vi "MQTT HASS Publisher.vi"() -> ()   [LabVIEW 2021]
uses:
  <vilib>/LabVIEW Open Source Project/MQTT Control Packets/Control Packets/CONNECT/ConnectFlags -- cluster.ctl
  <vilib>/LabVIEW Open Source Project/MQTT Connection/MQTT_Base/Base Class/MQTT_Base.lvclass/MQTT_Base.ctl
  <vilib>/LabVIEW Open Source Project/Connection/Connection.TCP/Connection.TCP.lvclass
  C:/Program Files (x86)/National Instruments/LabVIEW 2021/vi.lib/LabVIEW Open Source Project/Connection/Connection/Connection.lvclass
  <vilib>/LabVIEW Open Source Project/MQTT Client/Client class/Client.lvclass
  C:/Program Files (x86)/National Instruments/LabVIEW 2021/vi.lib/LabVIEW Open Source Project/MQTT Connection/MQTT_Base/Base Class/MQTT_Base.lvclass
  <vilib>/LabVIEW Open Source Project/MQTT Control Packets/Control Packets/PUBLISH/PUBLISH.lvclass
  <vilib>/LabVIEW Open Source Project/MQTT Connection/MQTT_Base/Base Class/MQTT_Base.lvclass
  <vilib>/LabVIEW Open Source Project/MQTT Control Packets/Control Packets/CONNECT/CONNECT.lvclass
  <vilib>/LabVIEW Open Source Project/MQTT Control Packets/Control Packets/ControlPacket/ControlPacket.lvclass
panel:
  out "Config Topic":string
  out "Voltage chart":dbl(graph)
  in  "Time Target (s)":dbl=0.5 format="%#_6ps"
  out "Current Chart":dbl(graph)
  out "State String":string
  out "Published State":bool
  in  "State topic":string="lab/psu/state"
  in  "Send Config Btn":bool
  out "Config String":string
  out "Connected?":bool
  out "Published Config":bool
  in  "remote port (1883)":u16=1883
  in  "address (localhost)":string="localhost"
  in  "STOP":bool
  # "HASS Publisher"
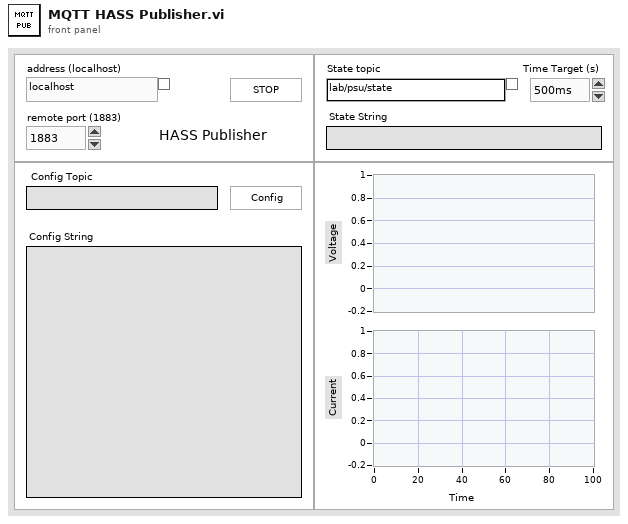
[diagram p1: front panel]
types:
  T1 = cluster{"Topic Name":string, "Config Message":string}[]
  T2 = enum32{"Invalid", "Standard", "Closed", "Hidden", "Minimized", "Maximized"}
  T3 = enum32{"invalid app kind", "Development System", "Run Time System", "Student Edition", "Embedded LabVIEW", "Evaluation", "Custom"}
  T4 = typedef "MQTT_Control_Packets.lvlib/CONNECT.lvclass/ConnectFlags -- cluster.ctl" = cluster{"Reserved":bool, "Clean Session":bool, "Will Flag":bool, "Will QoS 1":bool, "Will QoS 2":bool, "Will Retain":bool, "Password Flag":bool, "User Name Flag":bool}
  T5 = cluster{"Will Topic":string, "Will Message":string, "Username":string, "Password":string}
  T6 = cluster{"Core":cluster{"Current VI Reference":refnum<vi>, "Close Panel on Exit?":bool}, "Connected?":bool, "Published Config?":bool, "Published State?":bool, "Voltage":dbl, "Current":dbl}
  T7 = cluster{"Current VI Reference":refnum<vi>, "Close Panel on Exit?":bool}
  T8 = typedef "MQTT Base.lvlib/MQTT_Base.lvclass/Public Events -- cluster.ctl" = cluster{"Stop Event":refnum<user-event>, "Error Event":refnum<user-event>, "Inbound Message":refnum<user-event>}
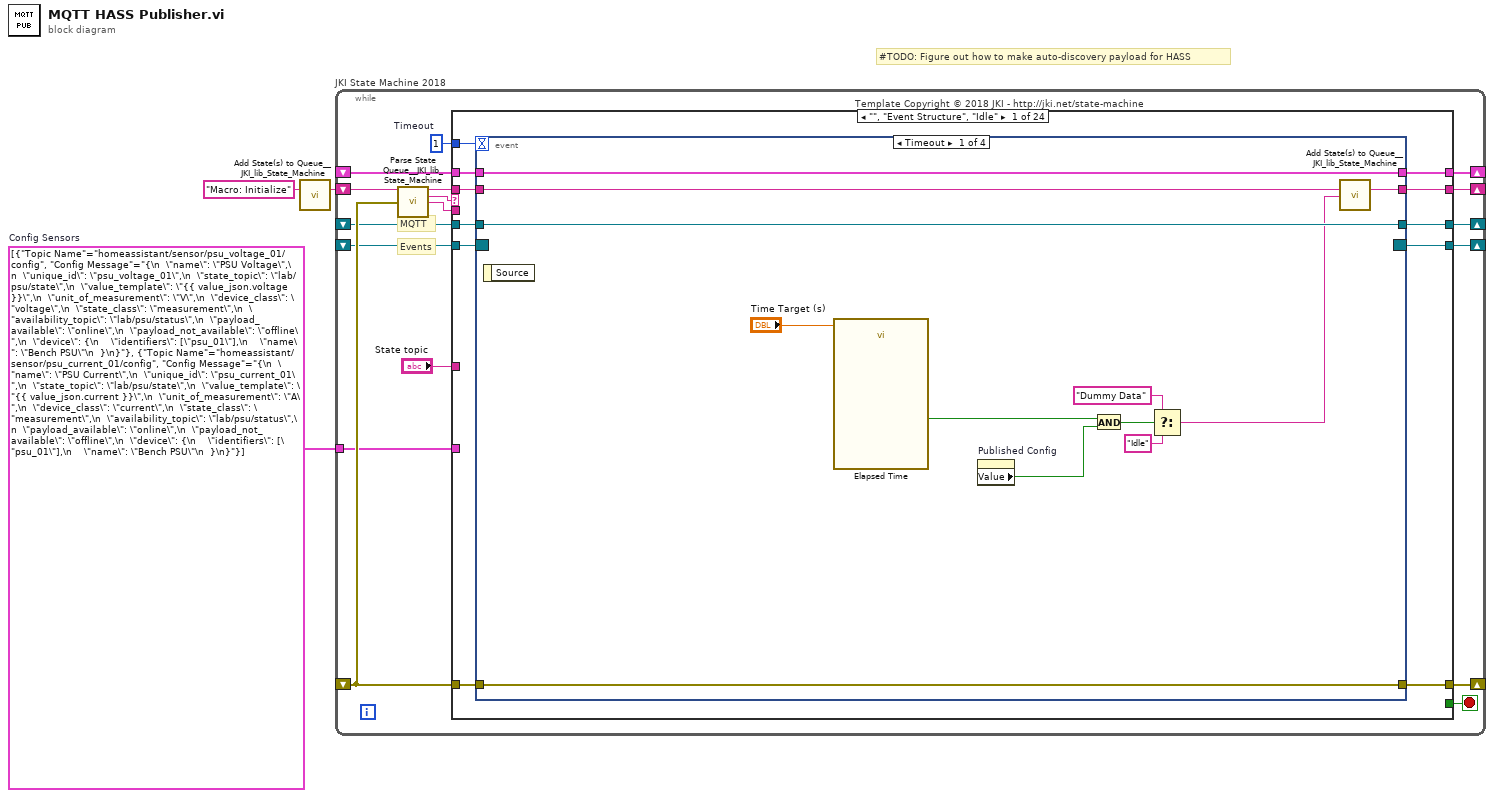
[diagram p0: block diagram]
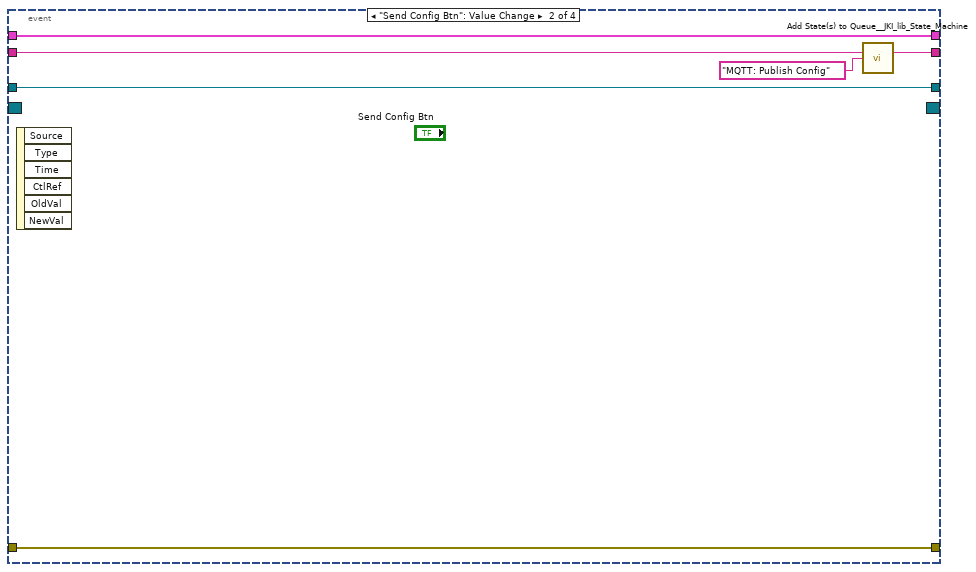
[diagram p2: hidden frame]
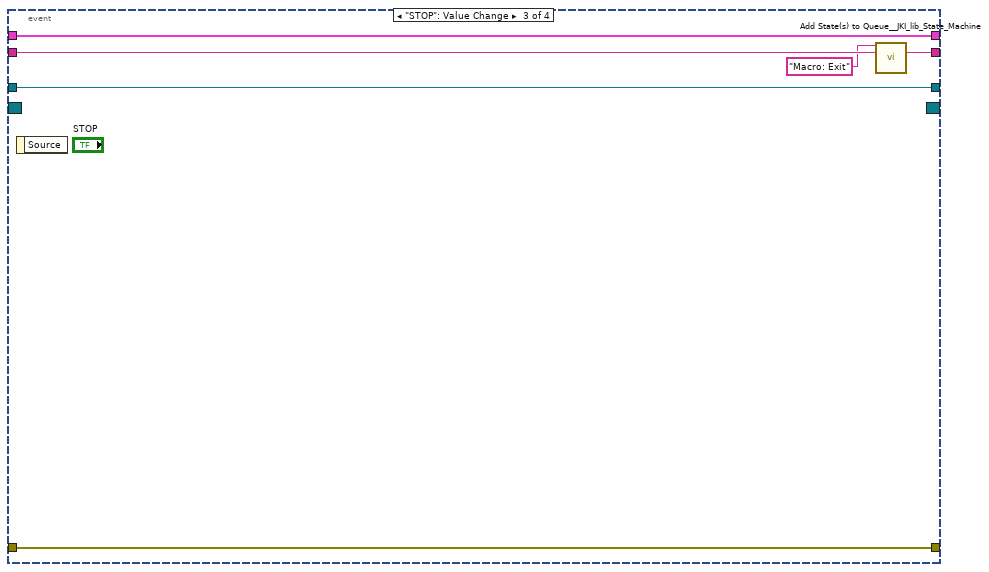
[diagram p3: hidden frame]
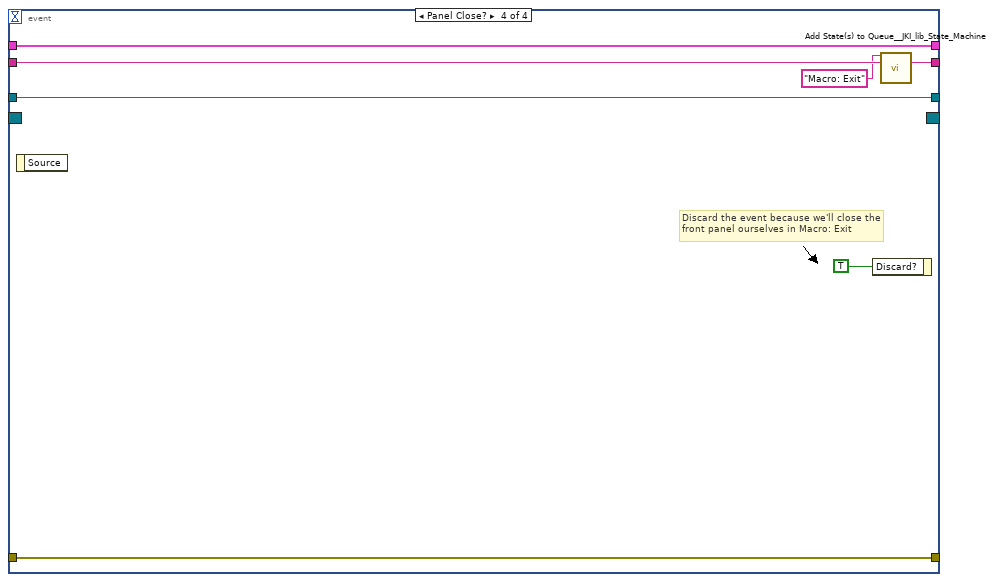
[diagram p4: hidden frame]
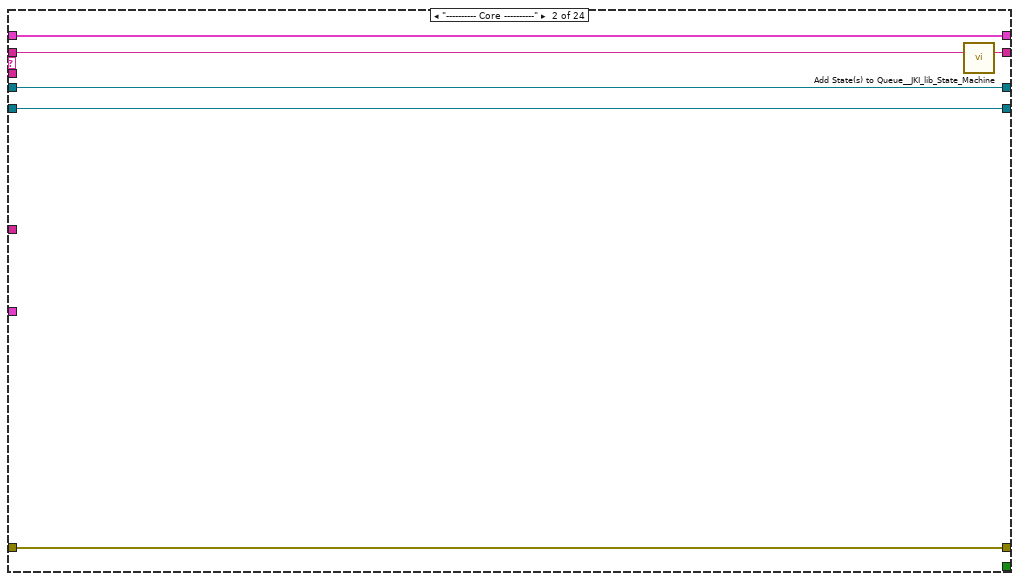
[diagram p5: hidden frame]
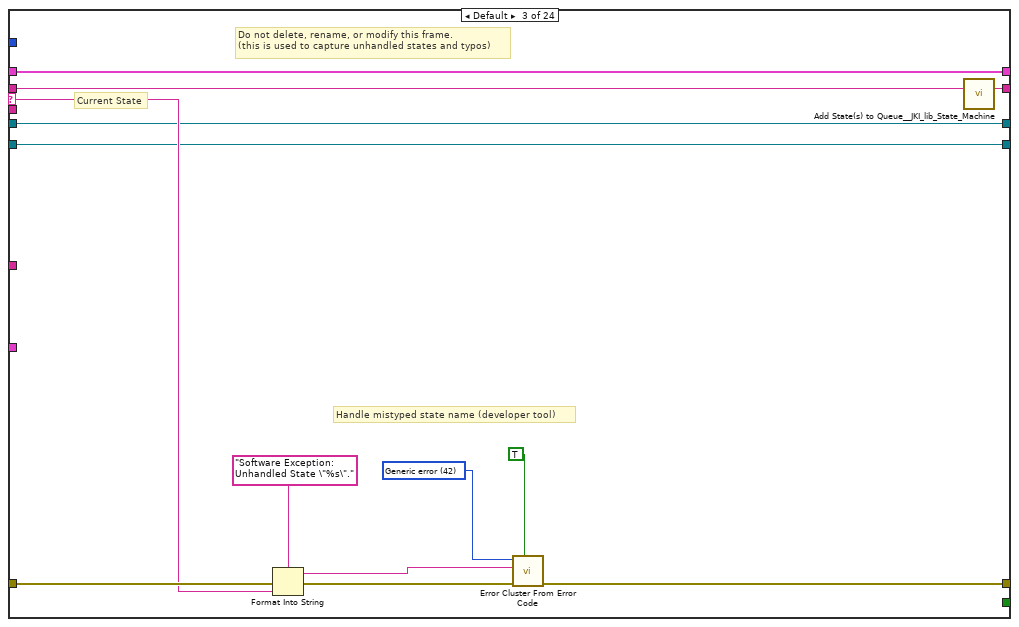
[diagram p6: hidden frame]
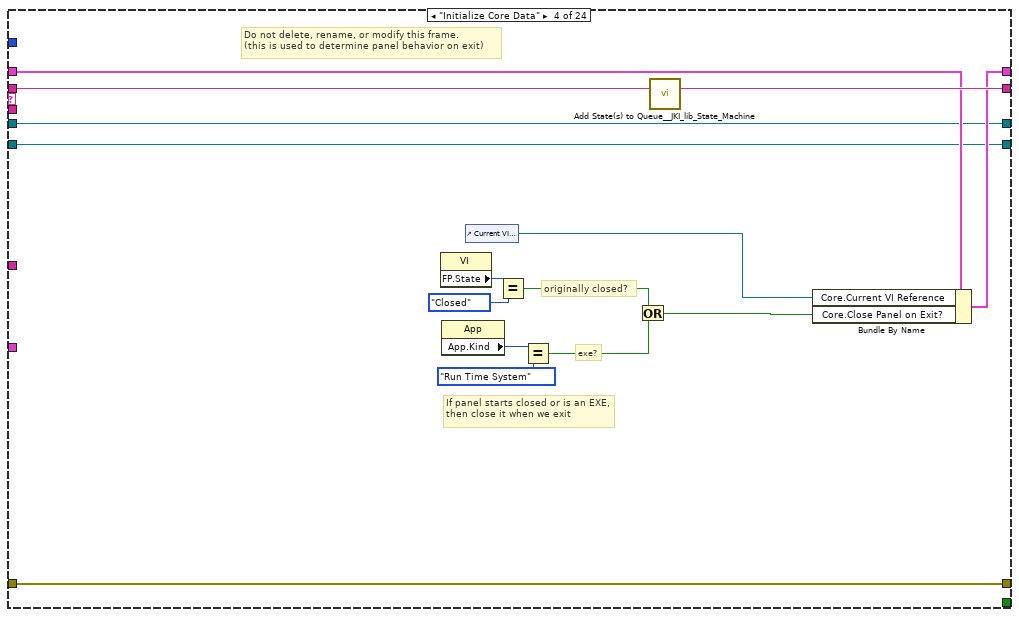
[diagram p7: hidden frame]
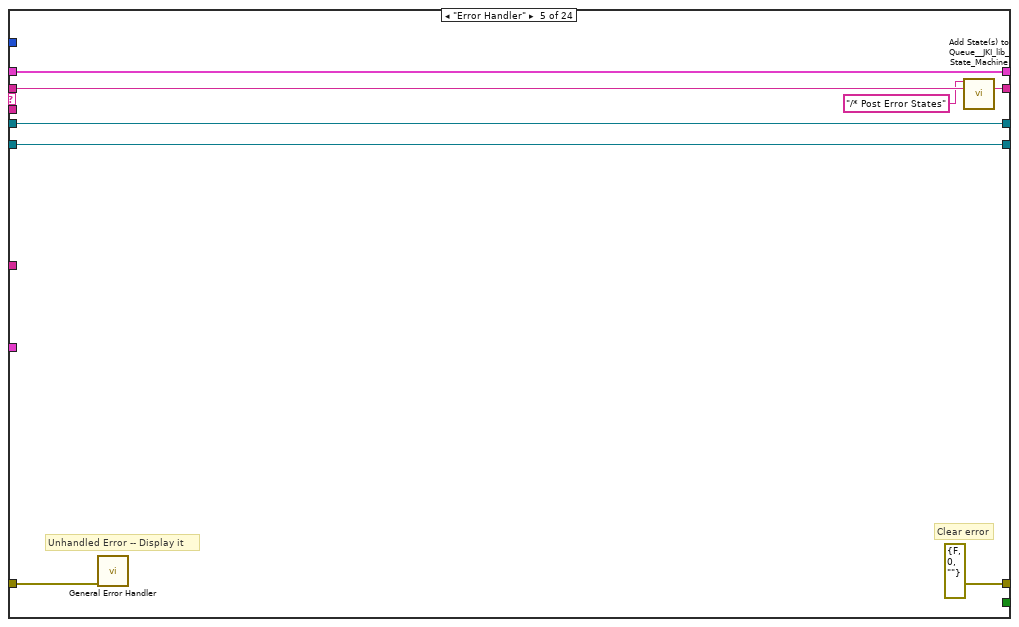
[diagram p8: hidden frame]
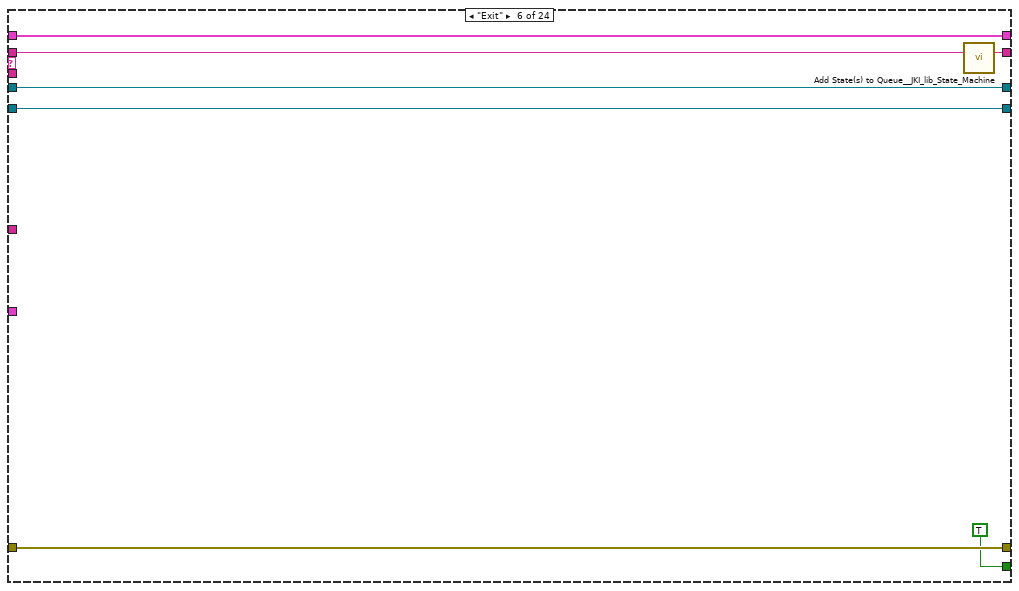
[diagram p9: hidden frame]
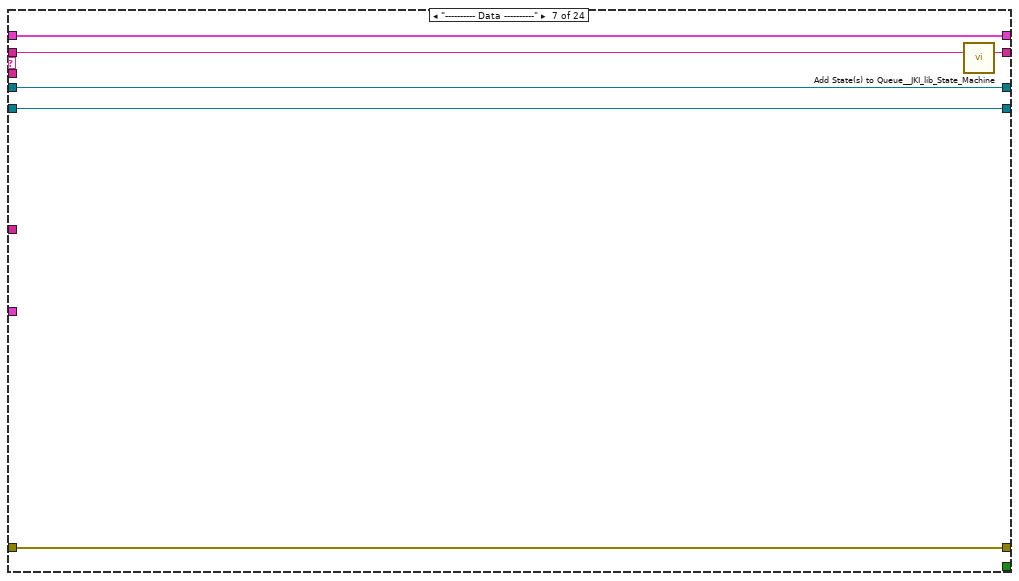
[diagram p10: hidden frame]
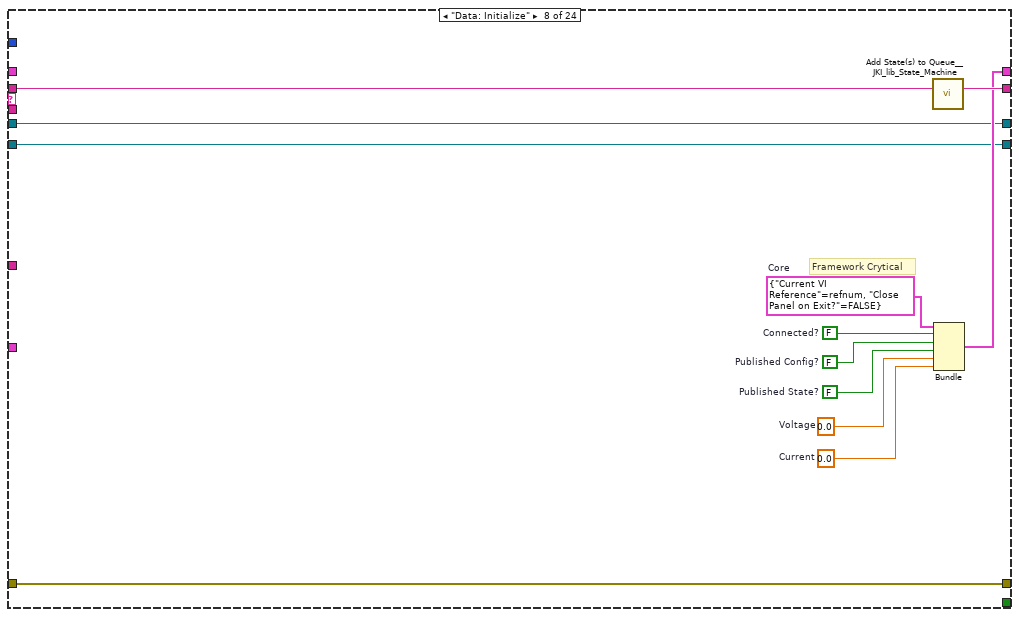
[diagram p11: hidden frame]
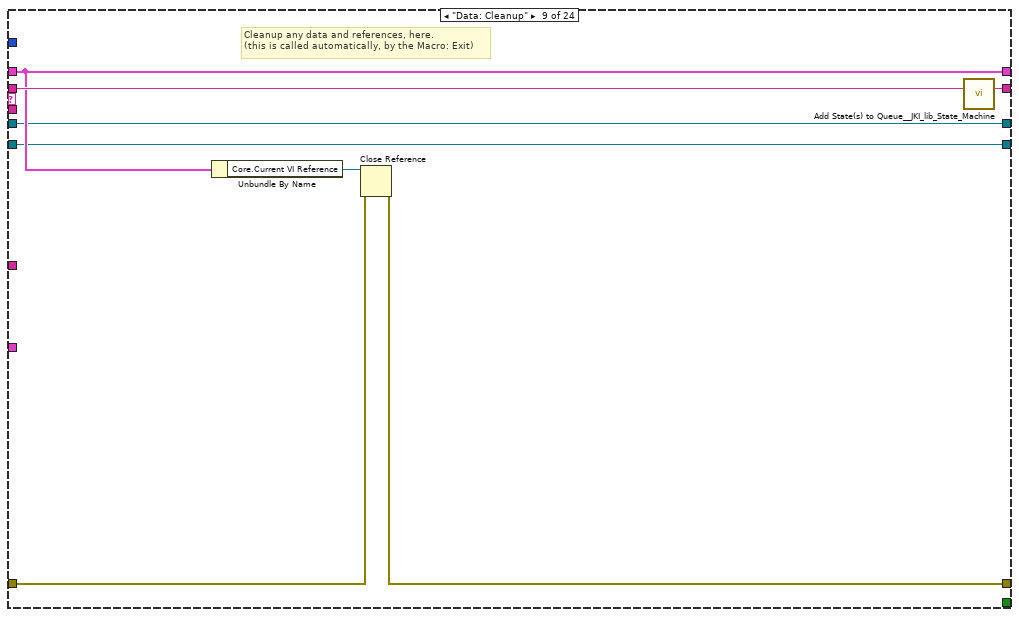
[diagram p12: hidden frame]
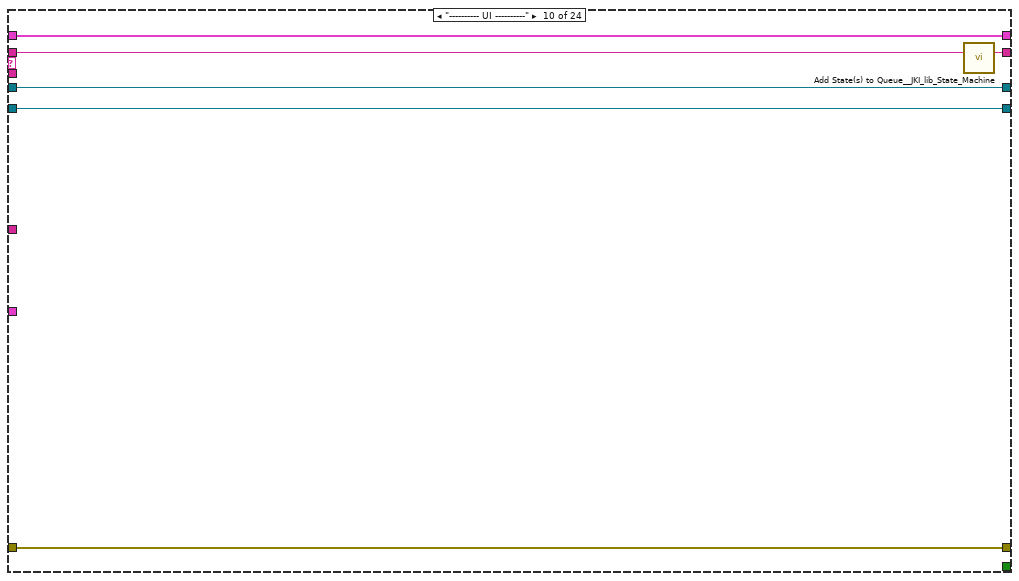
[diagram p13: hidden frame]
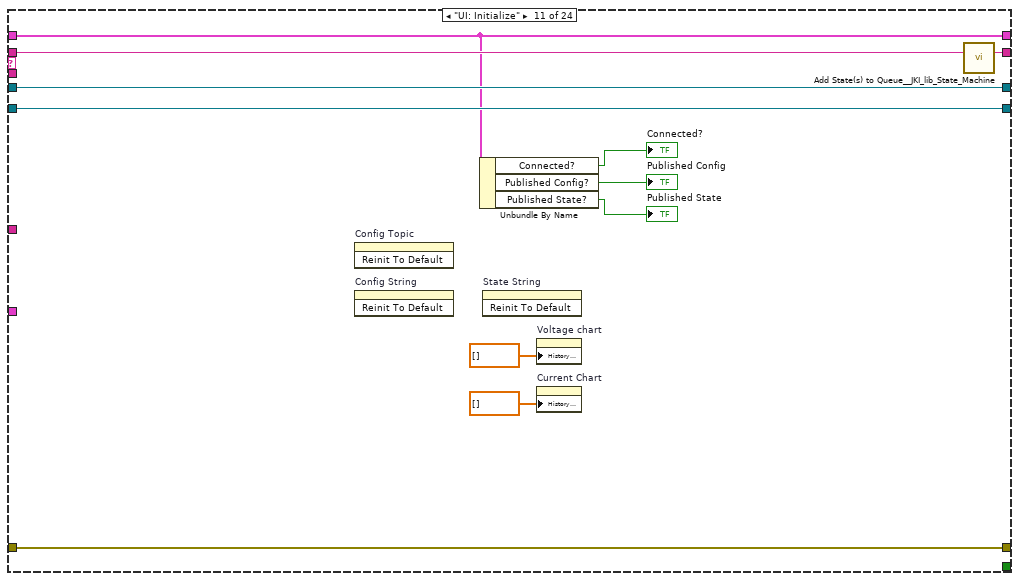
[diagram p14: hidden frame]
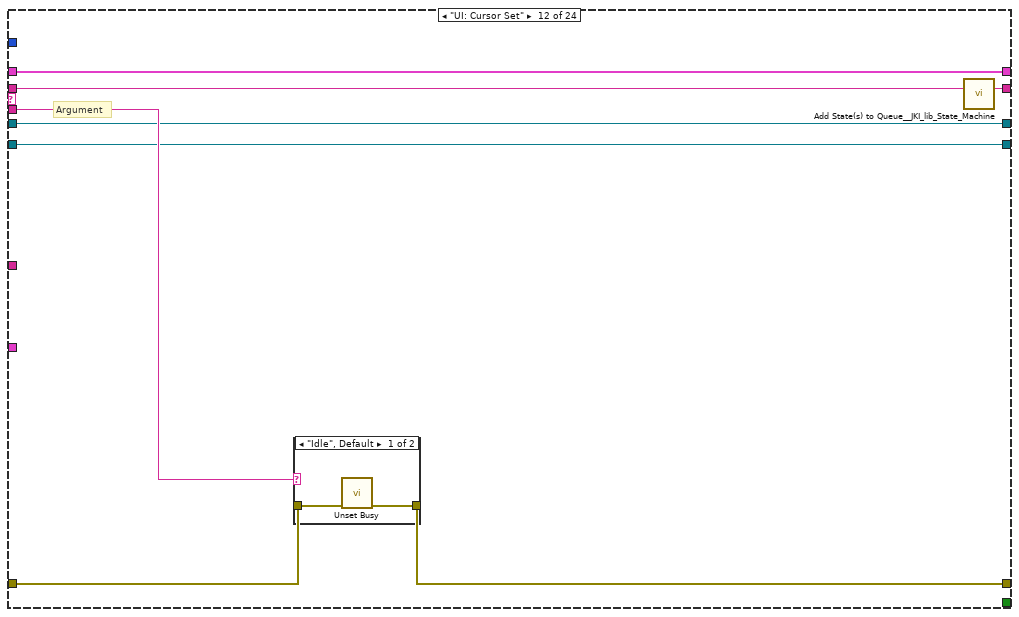
[diagram p15: hidden frame]
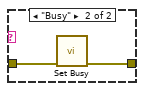
[diagram p16: hidden frame]
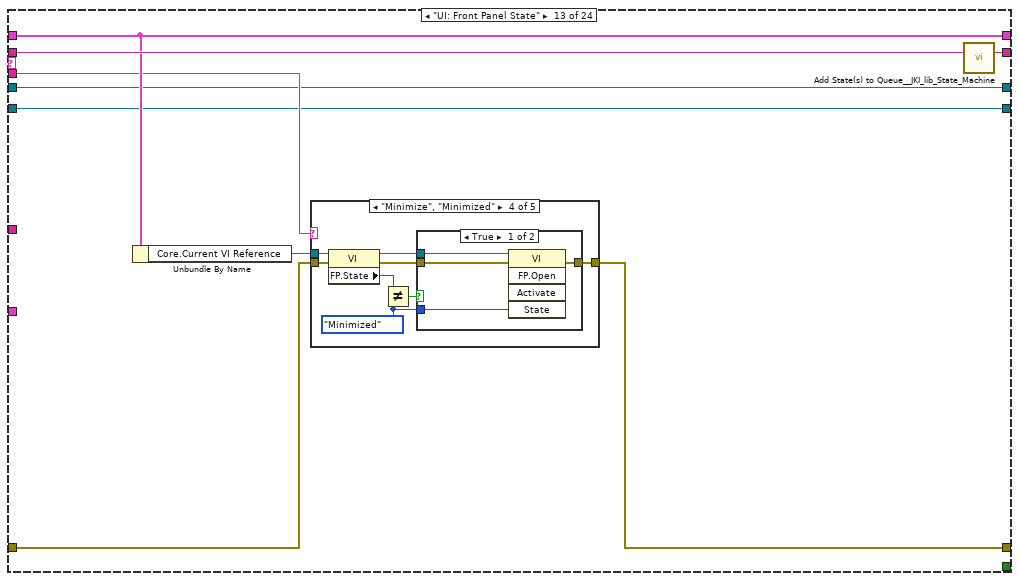
[diagram p17: hidden frame]
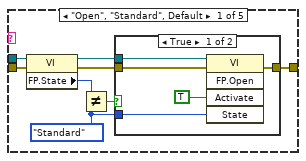
[diagram p18: hidden frame]
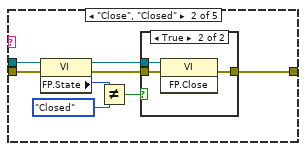
[diagram p20: hidden frame]
diagram:
  w1 = T1 [{"Topic Name"="homeassistant/sensor/psu_voltage_01/config", "Config Message"="{\n  \"name\": \"PSU Voltage\",\n  \"unique_id\": \"psu_voltage_01\",\n  \"state_topic\": \"lab/psu/state\",\n  \"value_template\": \"{{ value_json.voltage }}\",\n  \"unit_of_measurement\": \"V\",\n  \"device_class\": \"voltage\",\n  \"state_class\": \"measurement\",\n  \"availability_topic\": \"lab/psu/status\",\n  \"payload_available\": \"online\",\n  \"payload_not_available\": \"offline\",\n  \"device\": {\n    \"identifiers\": [\"psu_01\"],\n    \"name\": \"Bench PSU\"\n  }\n}"}, {"Topic Name"="homeassistant/sensor/psu_current_01/config", "Config Message"="{\n  \"name\": \"PSU Current\",\n  \"unique_id\": \"psu_current_01\",\n  \"state_topic\": \"lab/psu/state\",\n  \"value_template\": \"{{ value_json.current }}\",\n  \"unit_of_measurement\": \"A\",\n  \"device_class\": \"current\",\n  \"state_class\": \"measurement\",\n  \"availability_topic\": \"lab/psu/status\",\n  \"payload_available\": \"online\",\n  \"payload_not_available\": \"offline\",\n  \"device\": {\n    \"identifiers\": [\"psu_01\"],\n    \"name\": \"Bench PSU\"\n  }\n}"}]  # Config Sensors
  # "#TODO: Figure out how to make auto-discovery payload for HASS"
  n1 = call <vilib>:"Add State(s) to Queue__JKI_lib_State_Machine.vi"("State(s) in (\"\")"="Macro: Initialize") -> ("States Out"=w3:string)  [unwired: 14 in]
  n2 = while "JKI State Machine 2018" {
    shift-right: [w13] -> _
    shift-left: _ -> [w12]
    shift-right: [w16] -> _
    shift-left: _ -> [w10]
    shift-right: [w15] -> _
    shift-left: w3 -> [w17]
    shift-right: [w9] -> _
    shift-left: _ -> [w8]
    shift-right: [w7] -> _
    shift-left: _ -> [w6]
    tunnel: w1 -> [w4]
    stop <- w14 stop-if-true
    w11 = 1  # Timeout
    # "Events"
    # "MQTT"
    # "Template Copyright © 2018 JKI - http://jki.net/state-machine"
    n3 = call <vilib>:"Parse State Queue__JKI_lib_State_Machine.vi"("State Queue"=w17, "Error In (no error)"=w10) -> ("Remaining States"=w19:string, "Current State"=w20:string, "Arguments"=w18:string)  [unwired: 11 in]
    n4 = case shown="\"\", \"Event Structure\", \"Idle\"" w20 {
      selector: w20 -> [_ _ w71 _ _ _ _ _ _ _ _ _ _ _ _ _ _ _ _ _ _ _ _ _]
      tunnel: w19 -> [w31 w68 w75 w96 w104 w111 w117 w129 w137 w143 w154 w162 w175 w246 w253 w265 w271 w300 w315 w348 w377 w401 w415 w420]
      tunnel: w18 -> [_ _ _ _ _ _ _ _ _ _ _ w157 w169 _ _ _ _ _ _ _ _ _ _ _]
      tunnel: w12 -> [w29 w65 w73 w89 w101 w109 w114 _ w132 w140 w149 w160 w171 w243 w250 w262 w268 w280 w306 w336 w365 w389 w414 w423]
      tunnel: [w28 w66 w77 w93 errorcluster {"status"=FALSE, "code"=0, "source"=""} ("error out") w108 w115 w126 w133 w141 w152 w158 w172 w244 w251 w263 w269 w282 w308 w341 w370 w394 w416 w427] -> w16
      tunnel: w10 -> [w27 w66 w76 w93 w100 w108 w115 w126 w134 w141 w152 w159 w173 w244 w251 w263 w269 w298 w311 w344 w373 w397 w416 w427]
      tunnel: [w30 w67 w74 w95 w103 w110 w116 w128 w136 w142 w153 w161 w174 w245 w252 w264 w270 w299 w314 w347 w376 w400 w415 w421] -> w15
      tunnel: [_ _ _ _ _ TRUE _ _ _ _ _ _ _ _ _ _ _ _ _ _ _ _ _ _] -> w14
      tunnel: [w26 w65 w73 w94 w101 w109 w114 w127 w132 w140 w149 w160 w171 w243 w250 w262 w268 w279 w305 w339 w368 w392 w414 w422] -> w13
      tunnel: w11 -> [w25 _ _ _ _ _ _ _ _ _ _ _ _ _ _ _ _ _ _ _ _ _ _ _]
      tunnel: [w21 w63 w69 w82 w97 w105 w112 w123 w130 w138 w150 w155 w167 w241 w247 w254 w266 w297 w313 w346 w375 w399 w413 w426] -> w9
      tunnel: w8 -> [w22 w63 w69 w82 w97 w105 w112 w123 w130 w138 w150 w155 w167 w241 w247 w254 w266 _ w313 w346 w375 w399 w413 w426]
      tunnel: [w23 w64 w70 w83 w98 w106 w113 w124 w131 w139 w151 w156 w168 w242 w248 w255 w267 w281 w307 w340 w369 w393 w412 w425] -> w7
      tunnel: w6 -> [w24 w64 w70 w83 w98 w106 w113 w124 w131 w139 w151 w156 w168 w242 w248 w255 w267 _ w312 w345 w374 w398 w412 w425]
      tunnel: "State topic" -> [_ _ _ _ _ _ _ _ _ _ _ _ _ _ _ _ _ _ _ w335 w364 w388 _ _]
      tunnel: w4 -> [_ _ _ _ _ _ _ _ _ _ _ _ _ _ _ _ _ _ w301 _ _ _ _ _]
      frame "", "Event Structure", "Idle" {
        n5 = event shown="[0] Timeout" {
          selector: w22 -> [_ _ _ _]
          dyn-events: [_ _ _ _] -> w21
          timeout: w25 -> [_ _ _ _]
          tunnel: w31 -> [w43 w46 w55 w62]
          tunnel: [w42 w45 w54 w61] -> w30
          tunnel: w29 -> [w40 w48 w52 w59]
          tunnel: [w41 w49 w53 w60] -> w28
          tunnel: w27 -> [w41 w49 w53 w60]
          tunnel: [w40 w48 w52 w59] -> w26
          tunnel: w24 -> [w39 w47 w50 w56]
          tunnel: [w39 w47 w50 w56] -> w23
          event Timeout {
            n6 = event-data() -> ()  [unwired: 1 in, 1 out]
            n7 = call "Elapsed Time"("Time Target (s)"="Time Target (s)") -> ("Time has Elapsed"=w34:bool)  [unwired: 11 in, 7 out]
            n8 = property on="Published Config" class="Bool (strict)"() -> ("Value"=w33:bool)  [unwired: 2 in, 2 out]
            n9 = And(x=w34, y=w33) -> (x .and. y?=w32:bool)
            n10 = Select(t="Dummy Data" ("State(s) at Back (\"\")"), s=w32, f="Idle" ("State(s) at Back (\"\")")) -> (s? t:f=w35:string)
            n11 = call <vilib>:"Add State(s) to Queue__JKI_lib_State_Machine.vi"("State(s) in (\"\")"=w43, "State(s) at Back (\"\")"=w35) -> ("States Out"=w42:string)  [unwired: 13 in]
          }
          event "Send Config Btn": Value Change {
            n12 = event-data() -> ()  [unwired: 1 in, 6 out]
            n13 = call <vilib>:"Add State(s) to Queue__JKI_lib_State_Machine.vi"("State(s) in (\"\")"=w46, "State(s) at Back (\"\")"="MQTT: Publish Config" ("State(s) at Back (\"\")")) -> ("States Out"=w45:string)  [unwired: 13 in]
          }
          event "STOP": Value Change {
            n14 = event-data() -> ()  [unwired: 1 in, 1 out]
            n15 = call <vilib>:"Add State(s) to Queue__JKI_lib_State_Machine.vi"("State(s) in Front (\"\")"="Macro: Exit", "State(s) in (\"\")"=w55) -> ("States Out"=w54:string)  [unwired: 13 in]
          }
          event Panel Close? {
            # "Discard the event because we'll close the front panel ourselves in Macro: Exit"
            n16 = event-data() -> ()  [unwired: 1 in, 1 out]
            n17 = event-data("Discard?"=TRUE) -> ()  [unwired: 1 in, 1 out]
            n18 = call <vilib>:"Add State(s) to Queue__JKI_lib_State_Machine.vi"("State(s) in Front (\"\")"="Macro: Exit", "State(s) in (\"\")"=w62) -> ("States Out"=w61:string)  [unwired: 13 in]
          }
        }
      }
      frame "---------- Core ----------" {
        n19 = call <vilib>:"Add State(s) to Queue__JKI_lib_State_Machine.vi"("State(s) in (\"\")"=w68) -> ("States Out"=w67:string)  [unwired: 14 in]
      }
      frame Default {
        w80 = 42 items=["No error", "Argument error", "Memory is full", "Out of zone", "End of file", "File already open", "Generic file I/O error", "File not found", "File permission error", "Disk is full", "Duplicate path", "Too many files open", "System feature not enabled", "Resource file not found", "Cannot add resource", "Resource not found", "Image not found", "Image memory error", "Pen does not exist", "Config type invalid", "Config token not found", "Config parse error", "Config memory error", "Bad external code format", "Bad external code offset", "External code not present", "Null window", "Destroy window error", "Null menu", "Print aborted", "Bad print record", "Print driver error", "Windows error during printing", "Memory error during printing", "Print dialog error", "Generic print error", "Invalid device refnum", "Device not found", "Device parameter error", "Device unit error", "Cannot open device", "Device call aborted", "Generic error", "Cancelled by user", "Object ID too low", "Object ID too high", "Object not in heap", "Unknown heap", "Unknown object (invalid DefProc)", "Unknown object (DefProc not in table)", "Message out of range", "Invalid (null) method", "Unknown message", "Manager call not supported", "Bad address", "Network operation in progress", "Network operation timed out", "Connection is busy", "Network attribute not supported", "Network error", "Address in use", "System out of memory", "Connection aborted", "Connection refused", "Not connected", "Already connected", "Connection closed", "Initialization error (interapplication manager)", "Bad occurrence", "Wait on unbound occurrence handler", "Occurrence queue overflow", "Datalog type conflict", "Unused", "Unrecognized type (interapplication manager)", "Memory corrupt", "Failed to make temporary DLL", "Old CIN version", "Drag socket not found", "Failed to load drop-object", "Failed to register OLE object", "Failed to release OLE object", "Format specifier type mismatch", "Unknown format specifier", "Too few format specifiers", "Too many format specifiers", "Scan failed", "Newer CIN version", "Error converting to variant", "Runtime menu error", "Password tampered", "Variant attribute not found", "Incompatible variant data type", "Event data is not available", "Event Store is not present", "Occurrence is not found", "Event Queue is not created", "Event info is not available", "Refnum passed is NULL", "Error retrieving Class GUID", "Error retrieving CoClass GUID", "Error retrieving TypeLib GUID.", "Bad built application magic bytes.", "Specific driver is different from the specific driver associated with the Logical Name.", "There is no session opened to the class driver.", "Max Error", "MAX - Error with config objects", "MAX - Error loading configuration", "MAX - Group not supported"]
        # "Current State"
        # "Do not delete, rename, or modify this frame.\n(this is used to capture unhandled states and typos)"
        # "Handle mistyped state name (developer tool)"
        n20 = Format Into String(format string="Software Exception: Unhandled State \"%s\"." ("message"), error in=w76, w71) -> (resulting string=w79:string, error out=w78:errorcluster)  [unwired: 1 in]
        n21 = call <vilib>:"Error Cluster From Error Code.vi"("show call chain? (False)"=TRUE, "error in (no error)"=w78, "error message (\"\")"=w79, "error code (0)"=w80) -> ("error out"=w77:errorcluster)  [unwired: 5 in]
        n22 = call <vilib>:"Add State(s) to Queue__JKI_lib_State_Machine.vi"("State(s) in (\"\")"=w75) -> ("States Out"=w74:string)  [unwired: 14 in]
      }
      frame "Initialize Core Data" {
        # "Do not delete, rename, or modify this frame.\n(this is used to determine panel behavior on exit)"
        # "originally closed?"
        # "exe?"
        # "If panel starts closed or is an EXE, then close it when we exit"
        n23 = property class="VI"() -> ("FP.State"=w86:T2)  [unwired: 2 in, 2 out]
        n24 = property class="App"() -> ("App.Kind"=w92:T3)  [unwired: 2 in, 2 out]
        n25 = control-ref of="Current VI Reference"() -> (w87:refnum<vi>)
        n26 = Equal?(x=w86, y=T2."Closed" ("Front Panel Window:State")) -> (x = y?=w84:bool)
        n27 = Equal?(x=w92, y=T3."Run Time System" ("Application:Kind")) -> (x = y?=w90:bool)
        n28 = Or(x=w84, y=w90) -> (x .or. y?=w88:bool)
        n29 = call <vilib>:"Add State(s) to Queue__JKI_lib_State_Machine.vi"("State(s) in (\"\")"=w96) -> ("States Out"=w95:string)  [unwired: 14 in]
        n30 = Bundle By Name(cluster=w89, "Core.Current VI Reference"=w87, "Core.Close Panel on Exit?"=w88) -> (w94:T6)
      }
      frame "Error Handler" {
        # "Unhandled Error -- Display it"
        # "Clear error"
        n31 = call <vilib>:"General Error Handler.vi"("error in (no error)"=w100) -> ()  [unwired: 10 in, 5 out]
        n32 = call <vilib>:"Add State(s) to Queue__JKI_lib_State_Machine.vi"("State(s) in Front (\"\")"="/* Post Error States", "State(s) in (\"\")"=w104) -> ("States Out"=w103:string)  [unwired: 13 in]
      }
      frame "Exit" {
        n33 = call <vilib>:"Add State(s) to Queue__JKI_lib_State_Machine.vi"("State(s) in (\"\")"=w111) -> ("States Out"=w110:string)  [unwired: 14 in]
      }
      frame "---------- Data ----------" {
        n34 = call <vilib>:"Add State(s) to Queue__JKI_lib_State_Machine.vi"("State(s) in (\"\")"=w117) -> ("States Out"=w116:string)  [unwired: 14 in]
      }
      frame "Data: Initialize" {
        w118 = 0.0  # Current
        w119 = 0.0  # Voltage
        w120 = FALSE  # Published State?
        w121 = FALSE  # Published Config?
        w122 = FALSE  # Connected?
        w125 = T7 {"Current VI Reference"=refnum, "Close Panel on Exit?"=FALSE}  # Core
        # "Framework Crytical"
        n35 = call <vilib>:"Add State(s) to Queue__JKI_lib_State_Machine.vi"("State(s) in (\"\")"=w129) -> ("States Out"=w128:string)  [unwired: 14 in]
        n36 = Bundle("Core"=w125, "Connected?"=w122, "Published Config?"=w121, "Published State?"=w120, "Voltage"=w119, "Current"=w118) -> (w127:T6)  [unwired: 1 in]
      }
      frame "Data: Cleanup" {
        # "Cleanup any data and references, here.\n(this is called automatically, by the Macro: Exit)"
        n37 = Unbundle By Name(w132) -> ("Core.Current VI Reference"=w135:refnum<vi>)
        n38 = Close Reference(reference=w135, error in (no error)=w134) -> (error out=w133:errorcluster)
        n39 = call <vilib>:"Add State(s) to Queue__JKI_lib_State_Machine.vi"("State(s) in (\"\")"=w137) -> ("States Out"=w136:string)  [unwired: 14 in]
      }
      frame "---------- UI ----------" {
        n40 = call <vilib>:"Add State(s) to Queue__JKI_lib_State_Machine.vi"("State(s) in (\"\")"=w143) -> ("States Out"=w142:string)  [unwired: 14 in]
      }
      frame "UI: Initialize" {
        n41 = invoke on="Config Topic" class="Str" method="Reinit To Default"() -> ()  [unwired: 3 in, 3 out]
        n42 = invoke on="Config String" class="Str" method="Reinit To Default"() -> ()  [unwired: 3 in, 3 out]
        n43 = Unbundle By Name(w149) -> ("Connected?"=→"Connected?":bool, "Published Config?"=→"Published Config":bool, "Published State?"=→"Published State":bool)
        n44 = invoke on="State String" class="Str" method="Reinit To Default"() -> ()  [unwired: 3 in, 3 out]
        n45 = property on="Voltage chart" class="WFChart (strict)"("History Data"=dbl[] []) -> ()  [unwired: 2 in, 2 out]
        n46 = property on="Current Chart" class="WFChart (strict)"("History Data"=dbl[] []) -> ()  [unwired: 2 in, 2 out]
        n47 = call <vilib>:"Add State(s) to Queue__JKI_lib_State_Machine.vi"("State(s) in (\"\")"=w154) -> ("States Out"=w153:string)  [unwired: 14 in]
      }
      frame "UI: Cursor Set" {
        # "Argument"
        n48 = case shown="\"Idle\", Default" w157 {
          tunnel: w159 -> [w164 w166]
          tunnel: [w163 w165] -> w158
          frame "Idle", Default {
            n49 = call <vilib>:"Unset Busy.vi"("error in (no error)"=w164) -> ("error out"=w163:errorcluster)  [unwired: 10 in]
          }
          frame "Busy" {
            n50 = call <vilib>:"Set Busy.vi"("error in (no error)"=w166) -> ("error out"=w165:errorcluster)  [unwired: 9 in, 1 out]
          }
        }
        n51 = call <vilib>:"Add State(s) to Queue__JKI_lib_State_Machine.vi"("State(s) in (\"\")"=w162) -> ("States Out"=w161:string)  [unwired: 14 in]
      }
      frame "UI: Front Panel State" {
        n52 = Unbundle By Name(w171) -> ("Core.Current VI Reference"=w170:refnum<vi>)
        n53 = case shown="\"Minimize\", \"Minimized\"" w169 {
          tunnel: w173 -> [w181 w196 w207 w220 w233]
          tunnel: [w183 w197 w209 w222 w235] -> w172
          tunnel: w170 -> [w182 w194 w208 w221 w234]
          frame "Open", "Standard", Default {
            w176 = T2."Standard" ("State")
            n54 = property class="VI"(reference=w182, error in=w181) -> (reference out=w179:refnum<vi>, error out=w180:errorcluster, "FP.State"=w178:T2)
            n55 = Not Equal?(x=w178, y=w176) -> (x != y?=w177:bool)
            n56 = case shown="True" w177 {
              tunnel: [w187 w189] -> w183
              tunnel: w180 -> [w186 w189]
              tunnel: w179 -> [w185 _]
              tunnel: w176 -> [w184 _]
              frame True {
                n57 = invoke class="VI" method="FP.Open"(reference=w185, error in=w186, "Activate"=TRUE, "State"=w184) -> (error out=w187:errorcluster)  [unwired: 1 in, 4 out]
              }
              frame False {
              }
            }
          }
          frame "Close", "Closed" {
            n58 = property class="VI"(reference=w194, error in=w196) -> (reference out=w193:refnum<vi>, error out=w195:errorcluster, "FP.State"=w191:T2)
            n59 = Not Equal?(x=w191, y=T2."Closed" ("Front Panel Window:State")) -> (x != y?=w190:bool)
            n60 = case shown="True" w190 {
              tunnel: [w198 w201] -> w197
              tunnel: w195 -> [w198 w200]
              tunnel: w193 -> [_ w199]
              frame False {
              }
              frame True {
                n61 = invoke class="VI" method="FP.Close"(reference=w199, error in=w200) -> (error out=w201:errorcluster)  [unwired: 1 in, 2 out]
              }
            }
          }
          frame "Hidden", "Hide" {
            w202 = T2."Hidden" ("State")
            n62 = property class="VI"(reference=w208, error in=w207) -> (reference out=w205:refnum<vi>, error out=w206:errorcluster, "FP.State"=w204:T2)
            n63 = Not Equal?(x=w204, y=w202) -> (x != y?=w203:bool)
            n64 = case shown="True" w203 {
              tunnel: [w213 w214] -> w209
              tunnel: w206 -> [w212 w214]
              tunnel: w205 -> [w211 _]
              tunnel: w202 -> [w210 _]
              frame True {
                n65 = invoke class="VI" method="FP.Open"(reference=w211, error in=w212, "State"=w210) -> (error out=w213:errorcluster)  [unwired: 2 in, 4 out]
              }
              frame False {
              }
            }
          }
          frame "Minimize", "Minimized" {
            w215 = T2."Minimized" ("State")
            n66 = property class="VI"(reference=w221, error in=w220) -> (reference out=w218:refnum<vi>, error out=w219:errorcluster, "FP.State"=w217:T2)
            n67 = Not Equal?(x=w217, y=w215) -> (x != y?=w216:bool)
            n68 = case shown="True" w216 {
              tunnel: [w226 w227] -> w222
              tunnel: w219 -> [w225 w227]
              tunnel: w218 -> [w224 _]
              tunnel: w215 -> [w223 _]
              frame True {
                n69 = invoke class="VI" method="FP.Open"(reference=w224, error in=w225, "State"=w223) -> (error out=w226:errorcluster)  [unwired: 2 in, 4 out]
              }
              frame False {
              }
            }
          }
          frame "Maximize", "Maximized" {
            w228 = T2."Maximized" ("State")
            n70 = property class="VI"(reference=w234, error in=w233) -> (reference out=w231:refnum<vi>, error out=w232:errorcluster, "FP.State"=w230:T2)
            n71 = Not Equal?(x=w230, y=w228) -> (x != y?=w229:bool)
            n72 = case shown="True" w229 {
              tunnel: [w239 w240] -> w235
              tunnel: w232 -> [w238 w240]
              tunnel: w231 -> [w237 _]
              tunnel: w228 -> [w236 _]
              frame True {
                n73 = invoke class="VI" method="FP.Open"(reference=w237, error in=w238, "State"=w236) -> (error out=w239:errorcluster)  [unwired: 2 in, 4 out]
              }
              frame False {
              }
            }
          }
        }
        n74 = call <vilib>:"Add State(s) to Queue__JKI_lib_State_Machine.vi"("State(s) in (\"\")"=w175) -> ("States Out"=w174:string)  [unwired: 14 in]
      }
      frame "---------- Macro ----------" {
        n75 = call <vilib>:"Add State(s) to Queue__JKI_lib_State_Machine.vi"("State(s) in (\"\")"=w246) -> ("States Out"=w245:string)  [unwired: 14 in]
      }
      frame "Macro: Initialize" {
        n76 = call <vilib>:"Add State(s) to Queue__JKI_lib_State_Machine.vi"("State(s) in Front (\"\")"="Data: Initialize\nInitialize Core Data\nMQTT: Initialize\nUI: Initialize\nUI: Front Panel State >> Open", "State(s) in (\"\")"=w253) -> ("States Out"=w252:string)  [unwired: 13 in]
      }
      frame "Macro: Exit" {
        # "Signal the sensor is unavailable"
        n77 = Unbundle By Name(w262) -> ("Core.Close Panel on Exit?"=w261:bool)
        n78 = Select(t="UI: Front Panel State >> Close", s=w261, f="") -> (s? t:f=w258:string)
        n79 = call <vilib>:"Add State(s) to Queue__JKI_lib_State_Machine.vi"("State(s) in (\"\")"=w258, "State(s) at Back (\"\")"="MQTT: State Offline\nData: Cleanup\nExit") -> ("States Out"=w256:string)  [unwired: 13 in]
        n80 = call <vilib>:"Add State(s) to Queue__JKI_lib_State_Machine.vi"("State(s) in Front (\"\")"=w256, "State(s) in (\"\")"=w265) -> ("States Out"=w264:string)  [unwired: 13 in]
      }
      frame "---------- MQTT Broker ----------" {
        n81 = call <vilib>:"Add State(s) to Queue__JKI_lib_State_Machine.vi"("State(s) in (\"\")"=w271) -> ("States Out"=w270:string)  [unwired: 14 in]
      }
      frame "MQTT: Initialize" {
        w272 = FALSE ("Published?")
        # "Exit on fail"
        # "Connect"
        n82 = call <vilib>:"Configure TCP Connection.vi"("error in (no error)"=w298, "remote port (80)"="remote port (1883)", "address (localhost)"="address (localhost)") -> ("error out"=w293:errorcluster, "Connection.TCP"=w292:refnum<class "Connection.TCP.lvclass">)  [unwired: 7 in]
        n83 = call <vilib>:"Create MQTT Client.vi"("error in (no error)"=w293, "Connection Configuration"=w292) -> ("error out"=w290:errorcluster, "Client out"=w291:refnum<class "Client.lvclass">)  [unwired: 8 in]
        n84 = call <vilib>:"Read MQTT Public Events.vi"("error in (no error)"=w290, "MQTT_Base in"=w291) -> ("error out"=w288:errorcluster, "MQTT Public Events"=w289:T8, "MQTT_Base out"=w287:refnum<class "Client.lvclass">)  [unwired: 7 in]
        n85 = register-events(error in=w288, w289) -> (reference out=w297:refnum<event-registration>, error out=w296:errorcluster)  [unwired: 1 in]
        n86 = call <vilib>:"Start.vi"("error in (no error)"=w296, "MQTT_Base in"=w287) -> ("error out"=w285:errorcluster, "MQTT_Base out"=w286:refnum<class "Client.lvclass">)  [unwired: 7 in, 1 out]
        n87 = call <vilib>:"Connect to Server.vi"("Connect Flags"=T4 {"Reserved"=FALSE, "Clean Session"=TRUE, "Will Flag"=FALSE, "Will QoS 1"=FALSE, "Will QoS 2"=FALSE, "Will Retain"=FALSE, "Password Flag"=TRUE, "User Name Flag"=TRUE}, "Payload"=T5 {"Will Topic"="", "Will Message"="", "Username"="username", "Password"="password"}, "error in (no error)"=w285, "Client in"=w286) -> ("error out"=w283:errorcluster, "Client out"=w284:refnum<class "Client.lvclass">)  [unwired: 4 in, 2 out]
        n88 = call <vilib>:"isSessionConnected.vi"("error in (no error)"=w283, "MQTT_Base in"=w284) -> ("error out"=w282:errorcluster, "Connected?"=w278:bool, "MQTT_Base out"=w281:refnum<class "Client.lvclass">)  [unwired: 7 in]
        n89 = Bundle By Name(cluster=w280, "Connected?"=w278, "Published Config?"=w272, "Published State?"=w272) -> (w279:T6)
        n90 = Select(t="", s=w278, f="Macro: Exit" ("State(s) at Back (\"\")")) -> (s? t:f=w276:string)
        n91 = call <vilib>:"Add State(s) to Queue__JKI_lib_State_Machine.vi"("State(s) in (\"\")"=w300, "State(s) at Back (\"\")"=w276) -> ("States Out"=w299:string)  [unwired: 13 in]
      }
      frame "MQTT: Publish Config" {
        # "Signal the sensor is available"
        n92 = call <vilib>:"isSessionConnected.vi"("error in (no error)"=w311, "MQTT_Base in"=w312) -> ("error out"=w309:errorcluster, "Connected?"=w303:bool, "MQTT_Base out"=w310:refnum<class "Client.lvclass">)  [unwired: 7 in]
        n93 = property on="Connected?" class="Bool (strict)"("Value"=w303) -> ()  [unwired: 2 in, 2 out]
        n94 = for {
          shift-right: [w319] -> w307
          shift-left: w310 -> [w322]
          shift-right: [w320] -> w308
          shift-left: w309 -> [w321]
          tunnel: w303 -> [w317]
          tunnel: [w318] -> w304
          tunnel: w301 -> [w316] mode=indexing
          n95 = case shown="True" w317 {
            tunnel: w322 -> [w323 w330]
            tunnel: w321 -> [w324 w331]
            tunnel: [_ w333] -> w318
            tunnel: [w324 w332] -> w320
            tunnel: [w323 w334] -> w319
            tunnel: w316 -> [_ w328]
            frame False {
            }
            frame True {
              # "Wait so we can see what happens"
              n96 = Unbundle By Name(w328) -> ("Config Message"=w327:string)
              "Config String" <- w327
              n97 = Wait (ms)(milliseconds to wait=u32 1000) -> ()  [unwired: 1 out]
              n98 = Unbundle By Name(w328) -> ("Topic Name"=w325:string)
              "Config Topic" <- w325
              n99 = call <vilib>:"Encode TextString.vi"("Text String"=w327) -> ("Length-Prefixed Field"=w329:u8[])  [unwired: 10 in]
              n100 = call <vilib>:"Publish (Raw Payload).vi"("error in (no error)"=w331, "Binary Payload"=w329, "Topic Name"=w325, "Client in"=w330) -> ("error out"=w332:errorcluster, "Published"=w333:bool, "Client out"=w334:refnum<class "Client.lvclass">)  [unwired: 5 in]
            }
          }
        }
        n101 = Bundle By Name(cluster=w306, "Connected?"=w303, "Published State?"=w304) -> (w305:T6)
        n102 = property on="Published Config" class="Bool (strict)"("Value"=w304) -> ()  [unwired: 2 in, 2 out]
        n103 = call <vilib>:"Add State(s) to Queue__JKI_lib_State_Machine.vi"("State(s) in (\"\")"=w315, "State(s) at Back (\"\")"="MQTT: State Online" ("State(s) at Back (\"\")")) -> ("States Out"=w314:string)  [unwired: 13 in]
      }
      frame "MQTT: Publish State" {
        n104 = call <vilib>:"isSessionConnected.vi"("error in (no error)"=w344, "MQTT_Base in"=w345) -> ("error out"=w342:errorcluster, "Connected?"=w337:bool, "MQTT_Base out"=w343:refnum<class "Client.lvclass">)  [unwired: 7 in]
        n105 = property on="Connected?" class="Bool (strict)"("Value"=w337) -> ()  [unwired: 2 in, 2 out]
        n106 = case shown="True" w337 {
          tunnel: w343 -> [w349 w358]
          tunnel: w342 -> [w350 w359]
          tunnel: [_ w361] -> w338
          tunnel: [w350 w360] -> w341
          tunnel: [w349 w362] -> w340
          tunnel: w336 -> [_ w355]
          tunnel: w335 -> [_ w352]
          frame False {
          }
          frame True {
            n107 = Unbundle By Name(w355) -> ("Voltage"=w353:dbl, "Current"=w351:dbl)
            n108 = Format Into String(format string="{\"voltage\": %f, \"current\": %f}", w353, w351) -> (resulting string=w356:string)  [unwired: 2 in, 1 out]
            "State String" <- w356
            n109 = call <vilib>:"Encode TextString.vi"("Text String"=w356) -> ("Length-Prefixed Field"=w357:u8[])  [unwired: 10 in]
            n110 = call <vilib>:"Publish (Raw Payload).vi"("error in (no error)"=w359, "Binary Payload"=w357, "Topic Name"=w352, "Client in"=w358) -> ("error out"=w360:errorcluster, "Published"=w361:bool, "Client out"=w362:refnum<class "Client.lvclass">)  [unwired: 5 in]
          }
        }
        n111 = Bundle By Name(cluster=w336, "Connected?"=w337, "Published State?"=w338) -> (w339:T6)
        n112 = property on="Published State" class="Bool (strict)"("Value"=w338) -> ()  [unwired: 2 in, 2 out]
        n113 = call <vilib>:"Add State(s) to Queue__JKI_lib_State_Machine.vi"("State(s) in (\"\")"=w348) -> ("States Out"=w347:string)  [unwired: 14 in]
      }
      frame "MQTT: State Online" {
        # "Wait so we can see what happens"
        n114 = call <vilib>:"isSessionConnected.vi"("error in (no error)"=w373, "MQTT_Base in"=w374) -> ("error out"=w371:errorcluster, "Connected?"=w366:bool, "MQTT_Base out"=w372:refnum<class "Client.lvclass">)  [unwired: 7 in]
        n115 = property on="Connected?" class="Bool (strict)"("Value"=w366) -> ()  [unwired: 2 in, 2 out]
        n116 = case shown="True" w366 {
          tunnel: w372 -> [w378 w383]
          tunnel: w371 -> [w379 w384]
          tunnel: [_ w386] -> w367
          tunnel: [w379 w385] -> w370
          tunnel: [w378 w387] -> w369
          tunnel: w364 -> [_ w381]
          frame False {
          }
          frame True {
            w380 = "online" ("Text String")
            n117 = call <vilib>:"Encode TextString.vi"("Text String"=w380) -> ("Length-Prefixed Field"=w382:u8[])  [unwired: 10 in]
            n118 = property on="State String" class="Str"("Value"=w380) -> ()  [unwired: 2 in, 2 out]
            n119 = call <vilib>:"Publish (Raw Payload).vi"("error in (no error)"=w384, "Binary Payload"=w382, "Topic Name"=w381, "Client in"=w383) -> ("error out"=w385:errorcluster, "Published"=w386:bool, "Client out"=w387:refnum<class "Client.lvclass">)  [unwired: 5 in]
          }
        }
        n120 = Wait (ms)(milliseconds to wait=u32 1000) -> ()  [unwired: 1 out]
        n121 = Bundle By Name(cluster=w365, "Connected?"=w366, "Published State?"=w367) -> (w368:T6)
        n122 = property on="Published State" class="Bool (strict)"("Value"=w367) -> ()  [unwired: 2 in, 2 out]
        n123 = call <vilib>:"Add State(s) to Queue__JKI_lib_State_Machine.vi"("State(s) in (\"\")"=w377) -> ("States Out"=w376:string)  [unwired: 14 in]
      }
      frame "MQTT: State Offline" {
        n124 = call <vilib>:"isSessionConnected.vi"("error in (no error)"=w397, "MQTT_Base in"=w398) -> ("error out"=w395:errorcluster, "Connected?"=w390:bool, "MQTT_Base out"=w396:refnum<class "Client.lvclass">)  [unwired: 7 in]
        n125 = property on="Connected?" class="Bool (strict)"("Value"=w390) -> ()  [unwired: 2 in, 2 out]
        n126 = case shown="True" w390 {
          tunnel: w396 -> [w402 w407]
          tunnel: w395 -> [w403 w408]
          tunnel: [_ w410] -> w391
          tunnel: [w403 w409] -> w394
          tunnel: [w402 w411] -> w393
          tunnel: w388 -> [_ w405]
          frame False {
          }
          frame True {
            w404 = "offline" ("Text String")
            n127 = call <vilib>:"Encode TextString.vi"("Text String"=w404) -> ("Length-Prefixed Field"=w406:u8[])  [unwired: 10 in]
            n128 = property on="State String" class="Str"("Value"=w404) -> ()  [unwired: 2 in, 2 out]
            n129 = call <vilib>:"Publish (Raw Payload).vi"("error in (no error)"=w408, "Binary Payload"=w406, "Topic Name"=w405, "Client in"=w407) -> ("error out"=w409:errorcluster, "Published"=w410:bool, "Client out"=w411:refnum<class "Client.lvclass">)  [unwired: 5 in]
          }
        }
        n130 = Bundle By Name(cluster=w389, "Connected?"=w390, "Published State?"=w391) -> (w392:T6)
        n131 = property on="Published State" class="Bool (strict)"("Value"=w391) -> ()  [unwired: 2 in, 2 out]
        n132 = call <vilib>:"Add State(s) to Queue__JKI_lib_State_Machine.vi"("State(s) in (\"\")"=w401) -> ("States Out"=w400:string)  [unwired: 14 in]
      }
      frame "---------- Dummy Data ----------" {
      }
      frame "Dummy Data" {
        # "Generate a sine wave"
        n133 = for {
          N: 1 -> [_]
          shift-right: [w429] -> _
          shift-left: _ -> [w430]
          tunnel: [w432] -> w418
          tunnel: [w428] -> w417
          n134 = Add(x=0.1, y=w430) -> (x+y=w429:dbl)
          n135 = Sine(x=w429) -> (sin(x)=w432:dbl)
          n136 = Cosine(x=w429) -> (cos(x)=w428:dbl)
        }
        "Current Chart" <- w417
        "Voltage chart" <- w418
        n137 = Bundle By Name(cluster=w423, "Voltage"=w418, "Current"=w417) -> (w422:T6)
        n138 = call <vilib>:"Add State(s) to Queue__JKI_lib_State_Machine.vi"("State(s) in (\"\")"=w420, "State(s) at Back (\"\")"="MQTT: Publish State" ("State(s) at Back (\"\")")) -> ("States Out"=w421:string)  [unwired: 13 in]
      }
    }
  }
